vi "Initialize.vi"(8 "error in":errorcluster, 9 "Number of Channels":u32=1, 10 "Plugin Name":string, 11 "Power Supply in":refnum<class "Power Supply.lvclass">) -> (0 "error out":errorcluster, 3 "Power Supply out":refnum<class "Power Supply.lvclass">)   [LabVIEW 2023, in "Power Supply.lvclass"]
uses:
  Power Supply.lvclass
  Power Supply.lvclass/Power Supply.ctl
  <vilib>/ADAS Replay HIL/Channels/Tag Wrapper/Polymorphic/Open Producer Tag (Boolean).vi
  <vilib>/ADAS Replay HIL/Channels/Tag Wrapper/Polymorphic/Set Default Value (Boolean).vi
  <vilib>/ADAS Replay HIL/Channels/Tag Wrapper/Polymorphic/Open Producer Tag (Double).vi
  <vilib>/ADAS Replay HIL/Channels/Tag Wrapper/Polymorphic/Set Default Value (Double).vi
  <vilib>/ADAS Replay HIL/Channels/Tag Wrapper/Polymorphic/Open Producer Tag (Boolean).vi/45cd6eaa-a1ce-41a4-8aba-62a49d103d7e.vi
  <vilib>/ADAS Replay HIL/Channels/Tag Wrapper/Polymorphic/Set Default Value (Boolean).vi/228e99de-6fcf-414d-86fc-dc277c7b351f.vi
  <vilib>/ADAS Replay HIL/Channels/Tag Wrapper/Polymorphic/Open Producer Tag (Double).vi/45cd6eaa-a1ce-41a4-8aba-62a49d103d7e.vi
  <vilib>/ADAS Replay HIL/Channels/Tag Wrapper/Polymorphic/Set Default Value (Double).vi/228e99de-6fcf-414d-86fc-dc277c7b351f.vi
  <vilib>/ADAS Replay HIL/Channels/Tag Wrapper/Polymorphic/Open Producer Tag (Boolean).vi/45cd6eaa-a1ce-41a4-8aba-62a49d103d7e.vi/c28b0ead-42ad-4072-80a2-aca7f2bd7ce3.vi
  <vilib>/ADAS Replay HIL/Channels/Tag Wrapper/Polymorphic/Set Default Value (Boolean).vi/228e99de-6fcf-414d-86fc-dc277c7b351f.vi/4bc1c15b-36ab-481f-b8dd-c64075ce723a.vi
  <vilib>/ADAS Replay HIL/Channels/Tag Wrapper/Polymorphic/Open Producer Tag (Double).vi/45cd6eaa-a1ce-41a4-8aba-62a49d103d7e.vi/c28b0ead-42ad-4072-80a2-aca7f2bd7ce3.vi
  <vilib>/ADAS Replay HIL/Channels/Tag Wrapper/Polymorphic/Set Default Value (Double).vi/228e99de-6fcf-414d-86fc-dc277c7b351f.vi/4bc1c15b-36ab-481f-b8dd-c64075ce723a.vi
  <vilib>/ADAS Replay HIL/AdasHilServices/AdasHilServices Fill In Error Info Ex.vi
  Utilities/Utilities.lvlib
  <vilib>/ADAS Replay HIL/Channels/Tag Wrapper/Tag Wrapper.lvlib
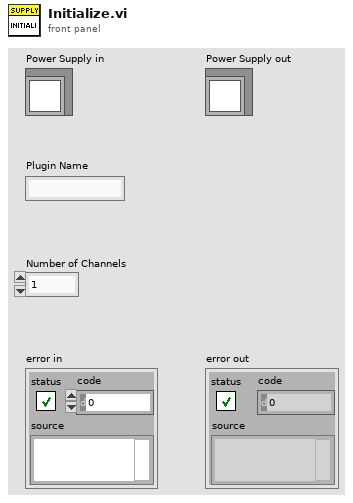
[diagram p1: front panel]
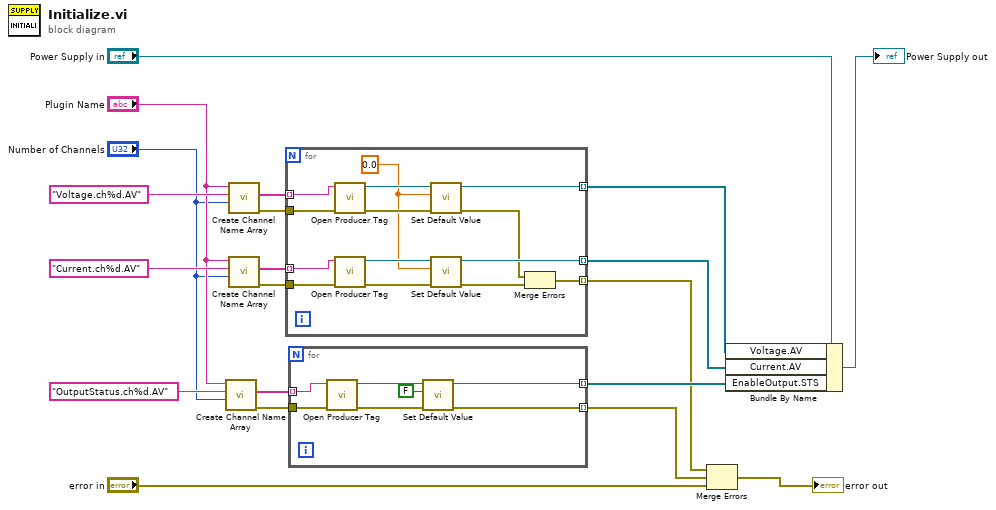
[diagram p0: block diagram]
diagram:
  n1 = call "Create Channel Name Array.vi"("Number of Channels"="Number of Channels", "Channel Format String"="OutputStatus.ch%d.AV", "Plugin Name"="Plugin Name") -> ("error out"=w8:errorcluster, "Channel Names"=w7:string[])  [unwired: 7 in]
  n2 = call "Create Channel Name Array.vi"("Number of Channels"="Number of Channels", "Channel Format String"="Voltage.ch%d.AV", "Plugin Name"="Plugin Name") -> ("error out"=w15:errorcluster, "Channel Names"=w16:string[])  [unwired: 7 in]
  n3 = call "Create Channel Name Array.vi"("Number of Channels"="Number of Channels", "Channel Format String"="Current.ch%d.AV", "Plugin Name"="Plugin Name") -> ("error out"=w13:errorcluster, "Channel Names"=w14:string[])  [unwired: 7 in]
  n4 = for {
    tunnel: w16 -> [w34] mode=indexing
    tunnel: [w32] -> w11 mode=indexing
    tunnel: w15 -> [w31]
    tunnel: w14 -> [w29] mode=indexing
    tunnel: w13 -> [w28]
    tunnel: [w26] -> w10 mode=indexing
    tunnel: [w21] -> w2 mode=indexing
    w24 = 0.0 ("Default Value")
    n5 = call-poly <vilib>:"Open Producer Tag.vi"("error in"=w31, "Channel Name"=w34) -> ("error out"=w30:errorcluster, "ADAS HIL Channel"=w33:refnum<k21>)  [unwired: 8 in]
    n6 = call-poly <vilib>:"Open Producer Tag.vi"("error in"=w28, "Channel Name"=w29) -> ("error out"=w25:errorcluster, "ADAS HIL Channel"=w27:refnum<k21>)  [unwired: 8 in]
    n7 = call-poly <vilib>:"Set Default Value.vi"("error in"=w30, "Default Value"=w24, "ADAS HIL Channel in"=w33) -> ("error out"=w23:errorcluster, "ADAS HIL Channel out"=w32:refnum<k21>)  [unwired: 7 in]
    n8 = call-poly <vilib>:"Set Default Value.vi"("error in"=w25, "Default Value"=w24, "ADAS HIL Channel in"=w27) -> ("error out"=w22:errorcluster, "ADAS HIL Channel out"=w26:refnum<k21>)  [unwired: 7 in]
    n9 = Merge Errors(w23, w22) -> (w21:errorcluster)
  }
  n10 = for {
    tunnel: w8 -> [w41]
    tunnel: w7 -> [w40] mode=indexing
    tunnel: [w35] -> w3 mode=indexing
    tunnel: [w36] -> w1 mode=indexing
    n11 = call-poly <vilib>:"Open Producer Tag.vi"("error in"=w41, "Channel Name"=w40) -> ("error out"=w38:errorcluster, "ADAS HIL Channel"=w39:refnum<k21>)  [unwired: 8 in]
    n12 = call-poly <vilib>:"Set Default Value.vi"("error in"=w38, "Default Value"=FALSE, "ADAS HIL Channel in"=w39) -> ("error out"=w36:errorcluster, "ADAS HIL Channel out"=w35:refnum<k21>)  [unwired: 7 in]
  }
  n13 = Merge Errors(w2, w1, "error in") -> (→"error out":errorcluster)
  n14 = Bundle By Name(cluster="Power Supply in", "Voltage.AV"=w11, "Current.AV"=w10, "EnableOutput.STS"=w3) -> (→"Power Supply out":refnum<class "Power Supply.lvclass">)
